vi "Translator.FormatMessage.vi"(9 "Arguments":variant[](array[variant]), 10 "Msg":string) -> (2 "Translated Msg":string)   [LabVIEW 2016]
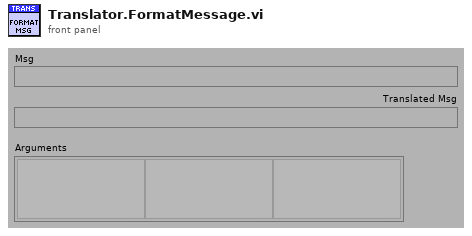
[diagram p1: front panel]
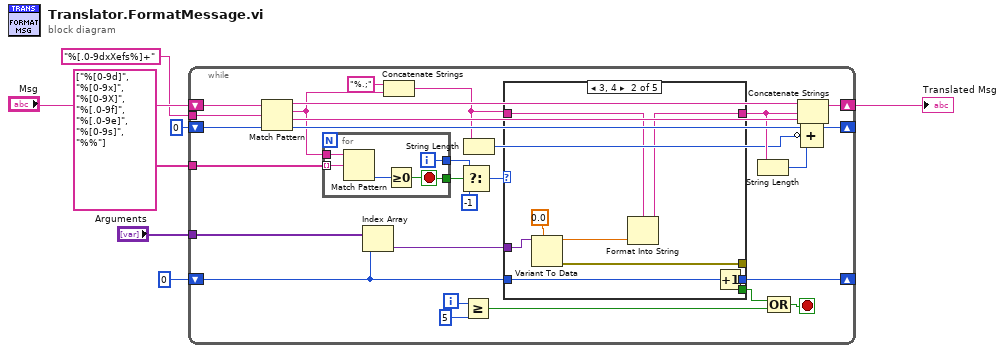
[diagram p0: block diagram]
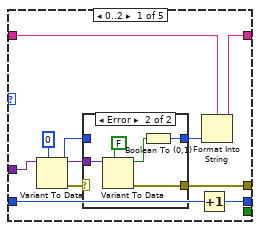
[diagram p2: hidden frame]
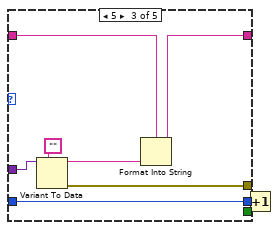
[diagram p4: hidden frame]
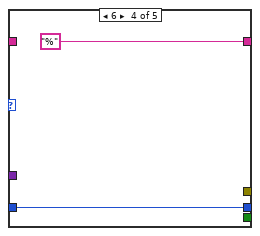
[diagram p5: hidden frame]
diagram:
  n1 = while {
    tunnel: string[] ["%[0-9d]", "%[0-9x]", "%[0-9X]", "%[.0-9f]", "%[.0-9e]", "%[0-9s]", "%%"] -> [w31]
    shift-right: [w35] -> _
    shift-left: 0 -> [w33]
    shift-right: [w15] -> _
    shift-left: 0 -> [w28]
    tunnel: "Arguments" -> [w34]
    shift-right: [w20] -> w7
    shift-left: "Msg" -> [w30]
    tunnel: "%[.0-9dxXefs%]+" -> [w29]
    i -> [w14]
    stop <- w19 stop-if-true
    n2 = Match Pattern(string=w30, regular expression=w29, offset (0)=w28) -> (before substring=w22:string, match substring=w10:string, after substring=w21:string, offset past match=w27:i32)
    n3 = for {
      tunnel: w10 -> [w77]
      tunnel: w31 -> [w76] mode=indexing
      tunnel: [w73] -> w24
      tunnel: [w74] -> w26
      i -> [w73]
      stop <- w74 stop-if-true
      n4 = Match Pattern(string=w77, regular expression=w76) -> (offset past match=w75:i32)  [unwired: 1 in, 3 out]
      n5 = Greater Or Equal To 0?(x=w75) -> (x >= 0?=w74:bool)
    }
    n6 = Index Array(array=w34, index=w33) -> (element=w32:variant)
    n7 = Concatenate Strings("%.;" ("string"), w10) -> (w8:string)
    n8 = Select(t=w24, s=w26, f=-1) -> (s? t:f=w25:i32)
    n9 = Greater Or Equal?(x=w14, y=5) -> (x >= y?=w12:bool)
    n10 = String Length(string=w8) -> (length=w17:i32)
    n11 = case shown="3, 4" w25 {
      tunnel: w33 -> [w42 w57 w67 w69 w72]
      tunnel: [w45 w60 w68 w69 w72] -> w35
      tunnel: w8 -> [w44 w59 w63 _ _]
      tunnel: w32 -> [w37 w55 w65 _ _]
      tunnel: [w41 w54 w61 "%" ("Msg") _] -> w18
      tunnel: [_ _ _ _ TRUE] -> w11
      tunnel: [w36 w53 w62 _ _] -> _
      frame 0..2 {
        n12 = Variant To Data(type=i64 0, Variant=w37) -> (data=w39:i64, error out=w40:errorcluster)  [unwired: 1 in]
        n13 = case shown="Error" w40 {
          selector: w40 -> [w47 _]
          tunnel: [w47 w50] -> w36
          tunnel: [w46 w48] -> w38
          tunnel: w39 -> [w46 _]
          tunnel: w37 -> [_ w51]
          frame No Error {
          }
          frame Error {
            n14 = Variant To Data(type=FALSE, Variant=w51) -> (data=w49:bool, error out=w50:errorcluster)  [unwired: 1 in]
            n15 = Boolean To (0,1)(Boolean=w49) -> (0, 1=w48:i16)
          }
        }
        n16 = Increment(x=w42) -> (x+1=w45:i32)
        n17 = Format Into String(format string=w44, w38) -> (resulting string=w41:string)  [unwired: 2 in, 1 out]
      }
      frame 3, 4 {
        n18 = Variant To Data(type=0.0, Variant=w55) -> (data=w56:dbl, error out=w53:errorcluster)  [unwired: 1 in]
        n19 = Format Into String(format string=w59, w56) -> (resulting string=w54:string)  [unwired: 2 in, 1 out]
        n20 = Increment(x=w57) -> (x+1=w60:i32)
      }
      frame 5 {
        n21 = Variant To Data(type="", Variant=w65) -> (data=w64:string, error out=w62:errorcluster)  [unwired: 1 in]
        n22 = Format Into String(format string=w63, w64) -> (resulting string=w61:string)  [unwired: 2 in, 1 out]
        n23 = Increment(x=w67) -> (x+1=w68:i32)
      }
      frame 6 {
      }
      frame Default {
      }
    }
    n24 = String Length(string=w18) -> (length=w16:i32)
    n25 = Compound Arithmetic op=OR(w11, w12) -> (w19:bool)
    n26 = Concatenate Strings(w22, w18, w21) -> (w20:string)
    n27 = Compound Arithmetic op=ADD(w27, invert w17, w16) -> (w15:i32)
  }
  "Translated Msg" <- w7
